vi "Get MCP Gain Table.vi"(9 "pfPhotoepc":sgl, 10 "piGain":i32, 11 "iNum":i32) -> (1 "pfPhotoepc out":sgl, 2 "piGain out":i32, 3 "function return":u32)   [LabVIEW 2018, in "Copy of Andor SDK.lvlib"]
doc: "EXPNETTYPE unsigned int WINAPI GetMCPGainTable(int iNum, int * piGain, float * pfPhotoepc);"
uses:
  Copy of Andor SDK.lvlib
  <userlib>/Andor SDK/ATMCD32D.dll
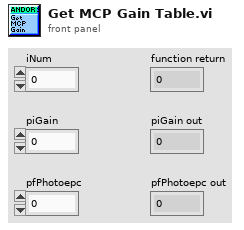
[diagram p1: front panel]
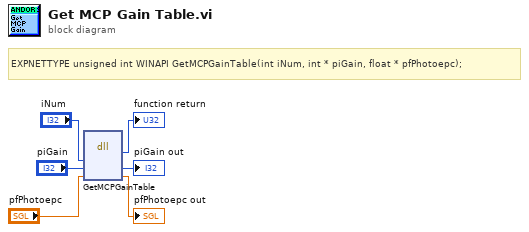
[diagram p0: block diagram]
diagram:
  # "EXPNETTYPE unsigned int WINAPI GetMCPGainTable(int iNum, int * piGain, float * pfPhotoepc);"
  n1 = dll-call lib="C:/Program Files (x86)/National Instruments/LabVIEW 2018/user.lib/Andor SDK/ATMCD32D.*" fn="GetMCPGainTable"("iNum"="iNum", "piGain"="piGain", "pfPhotoepc"="pfPhotoepc") -> (→"function return":u32, "piGain"=→"piGain out":i32, "pfPhotoepc"=→"pfPhotoepc out":sgl)  [unwired: 4 in, 2 out]
